vi "KListboxEx Test.vi"() -> ()   [LabVIEW 2020]
uses:
  KListboxEx/KListboxEx.xctl
panel:
  out "Event":string
  in  "stop":bool
  in  "KListboxEx":i32(xcontrol)
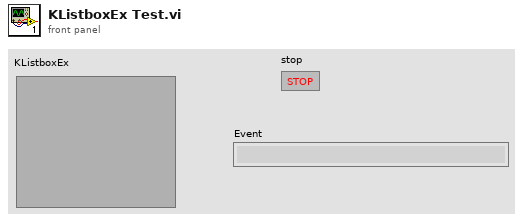
[diagram p1: front panel]
types:
  T1 = typedef "KListboxEx.xctl/Events.ctl" = cluster{"Items Changed":refnum<user-event>, "List Changed":refnum<user-event>}
  T2 = typedef "KListboxEx.xctl/Event Action.ctl" = enum16{"None", "Add", "Delete", "Move", "Edit", "Select"}
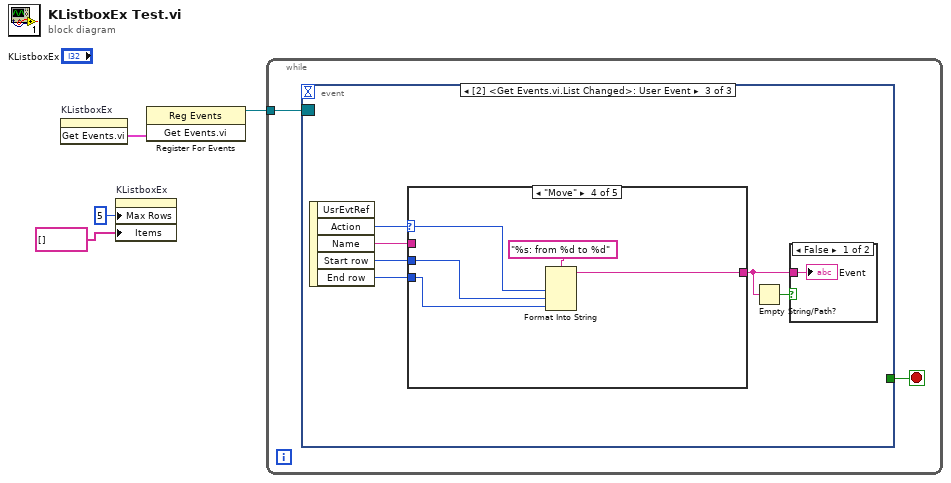
[diagram p0: block diagram]
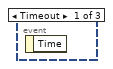
[diagram p2: hidden frame]
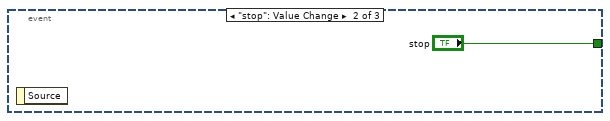
[diagram p3: hidden frame]
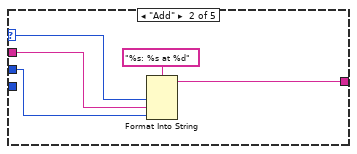
[diagram p6: hidden frame]
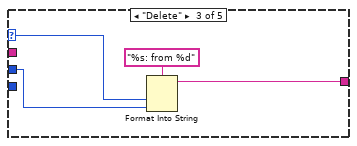
[diagram p7: hidden frame]
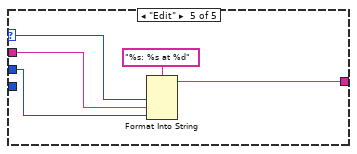
[diagram p8: hidden frame]
diagram:
  n1 = invoke on="KListboxEx" class="KListboxEx (strict)" method="Get Events.vi"() -> ("Get Events.vi"=w4:T1)  [unwired: 3 in, 2 out]
  n2 = property on="KListboxEx" class="KListboxEx (strict)"("Max Rows"=5, "Items"=string[] []) -> ()  [unwired: 2 in, 2 out]
  n3 = register-events(w4) -> (reference out=w3:refnum<event-registration>)  [unwired: 2 in, 1 out]
  n4 = while {
    tunnel: w3 -> [w5]
    stop <- w6 stop-if-true
    n5 = event shown="[2] <Get Events.vi.List Changed>: User Event" {
      selector: w5 -> [_ _ _]
      dyn-events: _ -> [_ _ _]
      timeout: _ -> [_ _ _]
      tunnel: [_ "stop" _] -> w6
      event Timeout {
        n6 = event-data() -> ()  [unwired: 1 in, 1 out]
      }
      event "stop": Value Change {
        n7 = event-data() -> ()  [unwired: 1 in, 1 out]
      }
      event User Event {
        n8 = event-data() -> ("Action"=w13:T2, "Name"=w12:string, "Start row"=w11:i32, "End row"=w10:i32)  [unwired: 1 in, 1 out]
        n9 = case shown="\"Move\"" w13 {
          selector: w13 -> [_ w18 w22 w27 w32]
          tunnel: w12 -> [_ w17 _ _ w31]
          tunnel: w11 -> [_ w16 w20 w25 w30]
          tunnel: w10 -> [_ _ _ w24 _]
          tunnel: [_ w15 w21 w26 w29] -> w9
          frame "None", Default {
          }
          frame "Add" {
            n10 = Format Into String(format string="%s: %s at %d", w18, w17, w16) -> (resulting string=w15:string)  [unwired: 2 in, 1 out]
          }
          frame "Delete" {
            n11 = Format Into String(format string="%s: from %d", w22, w20) -> (resulting string=w21:string)  [unwired: 2 in, 1 out]
          }
          frame "Move" {
            n12 = Format Into String(format string="%s: from %d to %d", w27, w25, w24) -> (resulting string=w26:string)  [unwired: 2 in, 1 out]
          }
          frame "Edit" {
            n13 = Format Into String(format string="%s: %s at %d", w32, w31, w30) -> (resulting string=w29:string)  [unwired: 2 in, 1 out]
          }
        }
        n14 = Empty String/Path?(string/path=w9) -> (empty?=w8:bool)
        n15 = case shown="False" w8 {
          tunnel: w9 -> [w14 _]
          frame False {
            "Event" <- w14
          }
          frame True {
          }
        }
      }
    }
  }
